vi "SPD.QE&TR Meas Const T.vi"(5 "Continue":refnum<vi>, 6 "Temperature index":i32, 7 "Progress":refnum<vi>, 8 "Error In":errorcluster, 10 "QEParams":T1, 11 "SPD.Stand Ctrl in":T2 {"spdDeviceSession"."hidSPD.Sturtup Values"."HV_bias" format="%#_6p, V"; "spdDeviceSession"."hidSPD.Sturtup Values"."TSet" format="%#_6p, DegC"; "spdDeviceSession"."hidSPD.Controller"."HV_bias" format="%#_6p, V"; "spdDeviceSession"."hidSPD.Controller"."TSet" format="%#_6p, DegC"}) -> (0 "Error Out":errorcluster, 1 "pass":bool, 2 "Report":string, 3 "SPD.Stand Ctrl out":T2 {"spdDeviceSession"."hidSPD.Sturtup Values"."HV_bias" format="%#_6p, V"; "spdDeviceSession"."hidSPD.Sturtup Values"."TSet" format="%#_6p, DegC"; "spdDeviceSession"."hidSPD.Controller"."HV_bias" format="%#_6p, V"; "spdDeviceSession"."hidSPD.Controller"."TSet" format="%#_6p, DegC"})   [LabVIEW 2018]
uses:
  typedefs/SPD.Stand Ctrl.ctl
  Instruments/SPD HID Interface/hidSPDLibForLabView/LibVIs/hidSPD Controls/hidSPD Device Session.ctl
  Instruments/SPD HID Interface/hidSPDLibForLabView/LibVIs/hidSPD Controls/hidSPD Controller.ctl
  Instruments/SPD HID Interface/hidSPDLibForLabView/LibVIs/hidSPD Controls/hidSPD SPD Type.ctl
  Instruments/KC705 DevBoard/typedefs/DevB.Session.ctl
  Instruments/KeySight 53230A/typedefs/FreqC.Session.ctl
  Instruments/KeySight 8164B/KeySight 8164B LAN InstrLib/typedefs/KeySight 8164B control.ctl
  Instruments/LeCroy SDA830/typedefs/LeCroy.Session.ctl
  typedefs/SPD.Events.ctl
  ConfigFile/SPD.Config File ctrl.ctl
  <vilib>/Utility/config.llb/Config Data RefNum.ctl
  typedefs/SPD.Meas Result.ctl
  typedefs/SPD.Queues.ctl
  typedefs/SPD.Stand state.ctl
  typedefs/SPD.QE Test Params.ctl
  typedefs/SPD.QE Strobe_Phase Tune Limits.ctl
  Instruments/KeySight 8164B/KeySight 8164B LAN InstrLib.lvlib
  <vilib>/Utility/config.llb/NI_LVConfig.lvlib
  Instruments/SPD HID Interface/hidSPDLibForLabView/hidSPDLibForLabView.lvlib
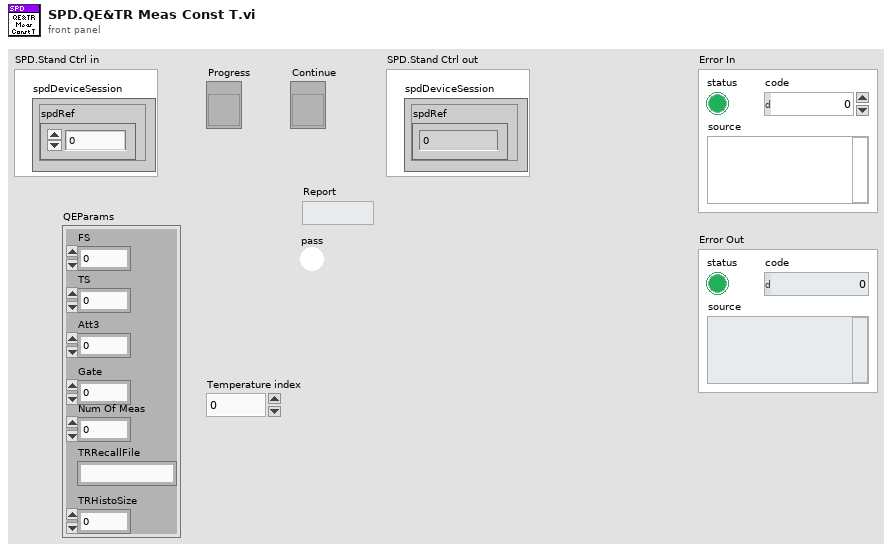
[diagram p1: front panel]
types:
  T1 = typedef "SPD.QE Test Params.ctl" = cluster{"FS":i32, "TS":i32, "Att3":dbl, "Gate":dbl, "Num Of Meas":i32, "TRRecallFile":string, "TRHistoSize":i32}
  T2 = typedef "SPD.Stand Ctrl.ctl" = cluster{"spdDeviceSession":T3, "DevBSession":T6, "FreqCSession":T7, "8164BSession":T8, "LeCroySession":T9, "Events":T10, "configFile":T11, "SPD.Result":T13, "SPD.Queues":T14, "Console":refnum<vi>}
  T3 = typedef "hidSPDLibForLabView.lvlib/hidSPD Device Session.ctl" = cluster{"spdRef":u64, "connected":bool, "spdName":string, "hidSPD.Controller":T4, "hidSPD.Sturtup Values":T4, "SPD Type":T5}
  T4 = typedef "hidSPDLibForLabView.lvlib/hidSPD Controller.ctl" = cluster{"TSet":sgl, "HV_bias":sgl, "DDS_stb_code":u16}
  T5 = typedef "hidSPDLibForLabView.lvlib/hidSPD SPD Type.ctl" = enum16{"Free Run", "Strobe"}
  T6 = typedef "DevB.Session.ctl" = cluster{"DevBRef":refnum<visa-resource-name>, "connected":bool}
  T7 = typedef "FreqC.Session.ctl" = cluster{"FreqCRef":refnum<visa-resource-name>, "timeout":dbl, "Gate":dbl, "connected":bool}
  T8 = typedef "KeySight 8164B LAN InstrLib.lvlib/KeySight 8164B control.ctl" = cluster{"Connection ID":refnum<k5>, "Connected":bool, "Info":string, "Slots Info":string[]}
  T9 = typedef "LeCroy.Session.ctl" = cluster{"LeCroySession":refnum<visa-resource-name>, "connected":bool}
  T10 = typedef "SPD.Events.ctl" = cluster{"DCRTest":refnum<user-event>, "Stop":refnum<user-event>}
  T11 = typedef "SPD.Config File ctrl.ctl" = cluster{"configFile ref":T12, "configFile path":path, "equipmentFile ref":T12}
  T12 = typedef "NI_LVConfig.lvlib/Config Data RefNum.ctl" = refnum<k1>
  T13 = typedef "SPD.Meas Result.ctl" = cluster{"HV_Bias":dbl[][][], "Stb_code":dbl[], "Temprature":dbl[], "Data":dbl[][][][], "DateTime":string}
  T14 = typedef "SPD.Queues.ctl" = cluster{"state queue":refnum<queue>}
  T15 = typedef "SPD.QE Strobe_Phase Tune Limits.ctl" = cluster{"ph_start":i32, "ph_stop":i32, "ph_step":i32}
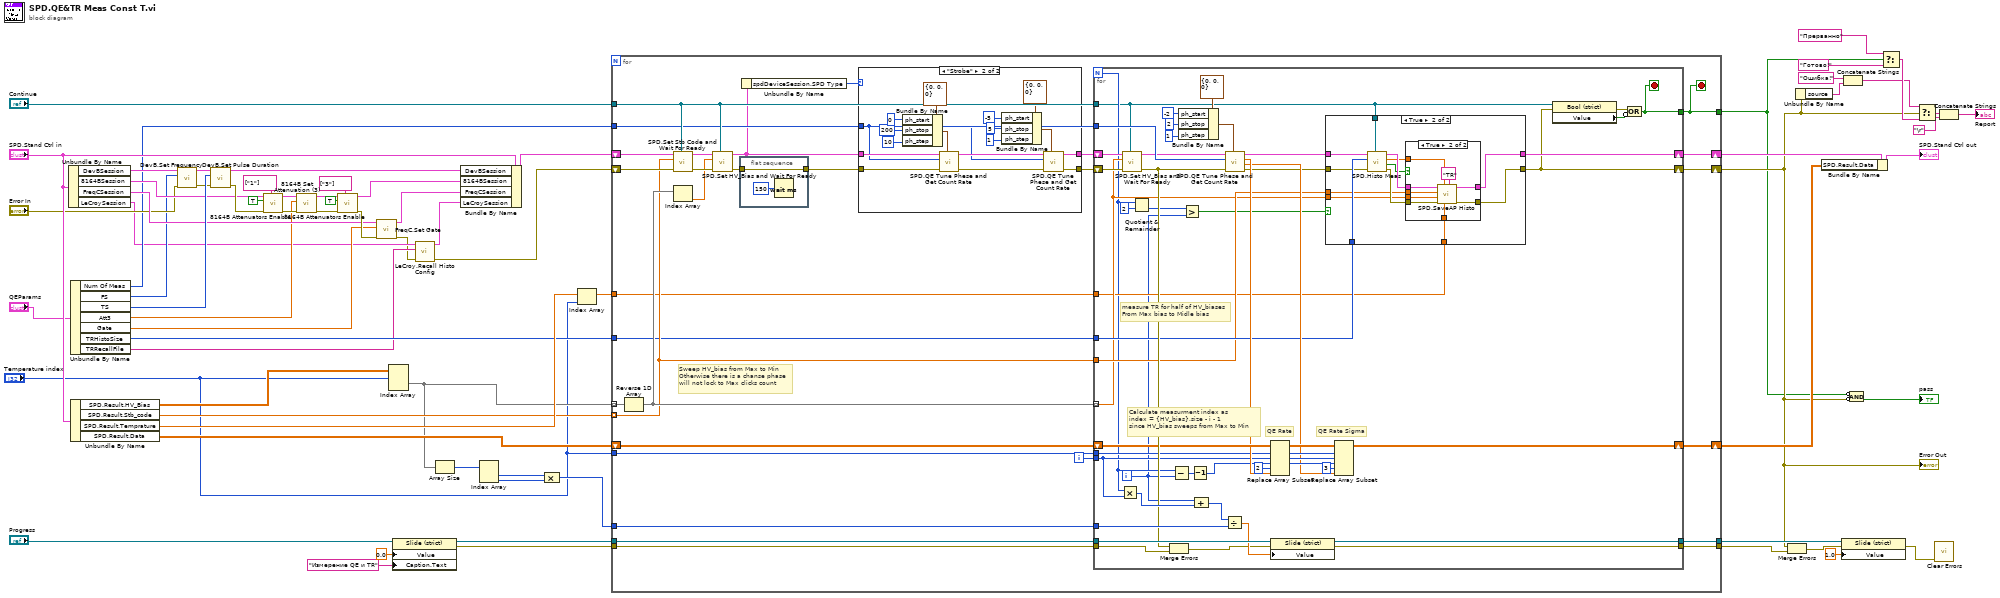
[diagram p0: block diagram]
diagram:
  n1 = Unbundle By Name("SPD.Stand Ctrl in") -> ("DevBSession"=w59:T6, "8164BSession"=w49:T8, "FreqCSession"=w48:T7, "LeCroySession"=w4:T9)
  n2 = Unbundle By Name("QEParams") -> ("Num Of Meas"=w32:i32, "FS"=w30:i32, "TS"=w57:i32, "Att3"=w31:dbl, "Gate"=w33:dbl, "TRHistoSize"=w17:i32, "TRRecallFile"=w5:string)
  n3 = Unbundle By Name("SPD.Stand Ctrl in") -> ("SPD.Result.HV_Bias"=w60:dbl[][][], "SPD.Result.Stb_code"=w61:dbl[], "SPD.Result.Temprature"=w62:dbl[], "SPD.Result.Data"=w41:dbl[][][][])
  n4 = call "DevB.Set Frequency.vi"("error in (no error)"="Error In", "Frequency"=w30, "DevB Session in"=w59) -> ("error out"=w56:errorcluster, "DevB Session out"=w58:T6)  [unwired: 7 in]
  n5 = call "DevB.Set Pulse Duration.vi"("error in (no error)"=w56, "Pulse Duration"=w57, "DevB Session in"=w58) -> ("error out"=w51:errorcluster, "DevB Session out"=w47:T6)  [unwired: 7 in]
  n6 = call "8164B Attenuators Enable.vi"("Slots"=string[] ["1"], "error in"=w51, "Enable"=TRUE, "KeySight 8164B control in"=w49) -> ("error out"=w35:errorcluster, "KeySight 8164B control out"=w37:T8)  [unwired: 6 in]
  n7 = call "8164B Set Attenuation (3).vi"("error in"=w35, "Att 3, dB"=w31, "KeySight 8164B control in"=w37) -> ("error out"=w34:errorcluster, "KeySight 8164B control out"=w36:T8)  [unwired: 7 in]
  n8 = call "8164B Attenuators Enable.vi"("Slots"=string[] ["3"], "error in"=w34, "Enable"=TRUE, "KeySight 8164B control in"=w36) -> ("error out"=w50:errorcluster, "KeySight 8164B control out"=w46:T8)  [unwired: 6 in]
  n9 = call "FreqC.Set Gate.vi"("error In"=w50, "Gate, sec"=w33, "FreqC Session in"=w48) -> ("error out"=w2:errorcluster, "FreqC Session out"=w45:T7)  [unwired: 7 in]
  n10 = Index Array(array=w60, index (dim 0)="Temperature index") -> (element=w15:dbl[][])  [unwired: 2 in]
  n11 = property class="Slide (strict)"(reference="Progress", "Value"=0.0, "Caption.Text"="Измерение QE и TR") -> (reference out=w11:refnum<vi>, error out=w9:errorcluster)  [unwired: 1 in]
  n12 = call "LeCroy.Recall Histo Config.vi"("Error In"=w2, "Filename (panel.lss)"=w5, "LeCroy.Session in"=w4) -> ("Error Out"=w1:errorcluster, "LeCroy.Session out"=w3:T9)  [unwired: 7 in]
  n13 = Array Size(array=w15) -> (size(s)=w40:i32[])
  n14 = Bundle By Name(cluster="SPD.Stand Ctrl in", "DevBSession"=w47, "8164BSession"=w46, "FreqCSession"=w45, "LeCroySession"=w3) -> (w16:T2)
  n15 = Index Array(array=w40) -> (element #1=w39:i32, element #2=w38:i32)  [unwired: 2 in]
  n16 = Compound Arithmetic op=MULTIPLY(w39, w38) -> (w66:i32)
  n17 = Index Array(array=w62, index="Temperature index") -> (element=w14:dbl)
  n18 = for {
    shift-right: [w98] -> w67
    shift-left: w41 -> [w100]
    tunnel: w15 -> [w85] mode=indexing
    tunnel: w61 -> [w77] mode=indexing
    shift-right: [w99] -> w70
    shift-left: w16 -> [w96]
    shift-right: [w97] -> w20
    shift-left: w1 -> [w95]
    tunnel: "Continue" -> [w86]
    tunnel: "Temperature index" -> [w94]
    tunnel: [w92] -> w19
    tunnel: w11 -> [w91]
    tunnel: w66 -> [w90]
    tunnel: [w89] -> w65
    tunnel: w32 -> [w81]
    tunnel: w17 -> [w76]
    tunnel: w14 -> [w75]
    tunnel: w9 -> [w74]
    tunnel: [w73] -> w7
    i -> [w93]
    stop <- w92 stop-if-true
    # "Sweep HV_bias from Max to Min\nOtherwise there is a chanse phase \nwill not lock to Max clicks count"
    n19 = Reverse 1D Array(array=w85) -> (reversed array=w78:dbl[])
    n20 = call "SPD.Set Stb Code and Wait For Ready.vi"("Continue"=w86, "Error In"=w95, "Strobe code"=w77, "SPD.Stand Ctrl in"=w96) -> ("Error Out"=w87:errorcluster, "SPD.Stand Ctrl out"=w88:T2)  [unwired: 6 in]
    n21 = Index Array(array=w78) -> (element=w84:dbl)  [unwired: 1 in]
    n22 = call "SPD.Set HV_Bias and Wait For Ready.vi"("Continue"=w86, "Error In"=w87, "HV_Bias"=w84, "SPD.Stand Ctrl in"=w88) -> ("Error Out"=w83:errorcluster, "SPD.Stand Ctrl out"=w72:T2)  [unwired: 6 in]
    n23 = flat-sequence {
      tunnel: w83 -> [w102]
      tunnel: [w102] -> w82
      frame #0 {
        n24 = Wait (ms)(milliseconds to wait=u32 150) -> ()  [unwired: 1 out]
      }
    }
    n25 = Unbundle By Name(w72) -> ("spdDeviceSession.SPD Type"=w71:T5)
    n26 = case shown="\"Strobe\"" w71 {
      tunnel: w82 -> [w103 w121]
      tunnel: w72 -> [w104 w120]
      tunnel: w81 -> [_ w107]
      tunnel: [w104 w106] -> w80
      tunnel: [w103 w105] -> w79
      frame "Free Run", Default {
      }
      frame "Strobe" {
        n27 = Bundle By Name(cluster=T15 {"ph_start"=0, "ph_stop"=0, "ph_step"=0} ("SPD.QE Strobe_Phase Tune Limits"), "ph_start"=0, "ph_stop"=200, "ph_step"=10) -> (w115:T15)
        n28 = call "SPD.QE Tune Phese and Get Count Rate.vi"("SPD.QE Strobe_Phase Tune Limits"=w115, "Error In"=w121, "Num of FreqC Meas"=w107, "SPD.Stand Ctrl in"=w120) -> ("Error Out"=w113:errorcluster, "SPD.Stand Ctrl out"=w114:T2)  [unwired: 4 in, 2 out]
        n29 = Bundle By Name(cluster=T15 {"ph_start"=0, "ph_stop"=0, "ph_step"=0} ("SPD.QE Strobe_Phase Tune Limits"), "ph_start"=-5, "ph_stop"=5, "ph_step"=1) -> (w108:T15)
        n30 = call "SPD.QE Tune Phese and Get Count Rate.vi"("SPD.QE Strobe_Phase Tune Limits"=w108, "Error In"=w113, "Num of FreqC Meas"=w107, "SPD.Stand Ctrl in"=w114) -> ("Error Out"=w105:errorcluster, "SPD.Stand Ctrl out"=w106:T2)  [unwired: 4 in, 2 out]
      }
    }
    n31 = for {
      N -> [w130]
      tunnel: w78 -> [w136] mode=indexing
      shift-right: [w143] -> w98
      shift-left: w100 -> [w153]
      shift-right: [w135] -> w99
      shift-left: w80 -> [w168]
      shift-right: [w134] -> w97
      shift-left: w79 -> [w167]
      tunnel: w86 -> [w122]
      tunnel: w94 -> [w142]
      tunnel: w93 -> [w141]
      tunnel: [w164] -> w92
      tunnel: w91 -> [w163]
      tunnel: w90 -> [w161]
      tunnel: [w159] -> w89
      tunnel: w81 -> [w156]
      tunnel: w77 -> [w137]
      tunnel: w76 -> [w138]
      tunnel: w75 -> [w133]
      tunnel: w74 -> [w124]
      tunnel: [w123] -> w73
      i -> [w127]
      stop <- w164 stop-if-true
      # "measure TR for half of HV_biases\nFrom Max bias to Midle bias"
      # "Calculate measurment index as \nindex = {HV_bias}.size - i - 1\nsince HV_bias sweeps from Max to Min"
      # "QE Rate Sigma"
      # "QE Rate"
      n32 = Multiply(x=w130, y=w141) -> (x*y=w157:i32)
      n33 = call "SPD.Set HV_Bias and Wait For Ready.vi"("Continue"=w122, "Error In"=w167, "HV_Bias"=w136, "SPD.Stand Ctrl in"=w168) -> ("Error Out"=w154:errorcluster, "SPD.Stand Ctrl out"=w155:T2)  [unwired: 6 in]
      n34 = Quotient & Remainder(x=w130, y=2) -> (floor(x/y)=w128:i32)  [unwired: 1 out]
      n35 = Merge Errors(w154, w124) -> (w125:errorcluster)
      n36 = Subtract(x=w130, y=w127) -> (x-y=w147:i32)
      n37 = Bundle By Name(cluster=T15 {"ph_start"=0, "ph_stop"=0, "ph_step"=0} ("SPD.QE Strobe_Phase Tune Limits"), "ph_start"=-2, "ph_stop"=2, "ph_step"=1) -> (w151:T15)
      n38 = Greater?(x=w128, y=w127) -> (0:w126:bool)
      n39 = Decrement(x=w147) -> (x-1=w140:i32)
      n40 = Compound Arithmetic op=ADD(w127, w157) -> (w162:i32)
      n41 = Divide(x=w162, y=w161) -> (x/y=w160:dbl)
      n42 = call "SPD.QE Tune Phese and Get Count Rate.vi"("SPD.QE Strobe_Phase Tune Limits"=w151, "Error In"=w154, "Num of FreqC Meas"=w156, "SPD.Stand Ctrl in"=w155) -> ("Error Out"=w131:errorcluster, "Count Sigma"=w139:dbl, "Count Rate"=w146:dbl, "SPD.Stand Ctrl out"=w132:T2)  [unwired: 4 in]
      n43 = Replace Array Subset(array=w153, new element=w146, index (dim 0)=w142, index (dim 1)=w141, index (dim 2)=w140, index (dim 3)=2 ("disabled index (col)")) -> (w144:dbl[][][][])
      n44 = property class="Slide (strict)"(reference=w163, error in=w125, "Value"=w160) -> (reference out=w159:refnum<vi>, error out=w123:errorcluster)
      n45 = case shown="True" w126 {
        tunnel: w132 -> [w170 w183]
        tunnel: w138 -> [_ w182]
        tunnel: w131 -> [w169 w181]
        tunnel: w137 -> [_ w178]
        tunnel: w136 -> [_ w177]
        tunnel: [w170 w176] -> w135
        tunnel: [w169 w175] -> w134
        tunnel: w133 -> [_ w174]
        tunnel: w122 -> [_ w173]
        frame False {
        }
        frame True {
          n46 = call "SPD.Histo Meas.vi"("Continue"=w173, "Error In"=w181, "Histo length"=w182, "SPD.Stand Ctrl in"=w183) -> ("Error Out"=w179:errorcluster, "pass"=w172:bool, "AP Histo"=w171:dbl[], "SPD.Stand Ctrl out"=w180:T2)  [unwired: 4 in]
          n47 = case shown="True" w172 {
            tunnel: w180 -> [w185 w194]
            tunnel: w179 -> [w184 w193]
            tunnel: w178 -> [_ w192]
            tunnel: w177 -> [_ w191]
            tunnel: [w185 w189] -> w176
            tunnel: [w184 w188] -> w175
            tunnel: w174 -> [_ w187]
            tunnel: w171 -> [_ w186]
            frame False {
            }
            frame True {
              n48 = call "SPD.SaveAP Histo.vi"("Name"="TR", "Temperature"=w187, "AP Histo"=w186, "Error In"=w193, "HV_bias"=w191, "Stb_Code"=w192, "SPD.Stand Ctrl in"=w194) -> ("Error Out"=w188:errorcluster, "SPD.Stand Ctrl out"=w189:T2)  [unwired: 3 in]
            }
          }
        }
      }
      n49 = Replace Array Subset(array=w144, new element=w139, index (dim 0)=w142, index (dim 1)=w141, index (dim 2)=w140, index (dim 3)=3 ("disabled index (col)")) -> (w143:dbl[][][][])
      n50 = property class="Bool (strict)"(reference=w122, error in=w134) -> (error out=w165:errorcluster, "Value"=w166:bool)  [unwired: 1 out]
      n51 = Compound Arithmetic op=OR(w165, invert w166) -> (w164:bool)
    }
  }
  "Error Out" <- w20
  n52 = Merge Errors(w20, w7) -> (w8:errorcluster)
  n53 = Unbundle By Name(w20) -> ("source"=w25:string)
  n54 = Bundle By Name(cluster=w70, "SPD.Result.Data"=w67) -> (→"SPD.Stand Ctrl out":T2)
  n55 = property class="Slide (strict)"(reference=w65, error in=w8, "Value"=1.0) -> (error out=w63:errorcluster)  [unwired: 1 out]
  n56 = Concatenate Strings("Ошибка!" ("t"), w25) -> (w26:string)
  n57 = Compound Arithmetic op=AND(invert w19, invert w20) -> (→"pass":bool)
  n58 = Select(t="Прерванно" ("Report"), s=w19, f="Готово!") -> (s? t:f=w28:string)
  n59 = Select(t=w26, s=w20, f=w28) -> (s? t:f=w23:string)
  n60 = call <vilib>:"Clear Errors.vi"("error in (no error)"=w63) -> ()  [unwired: 5 in, 2 out]
  n61 = Concatenate Strings(w23, "\r") -> (→"Report":string)
